vi "test write exist frame.vi"() -> ()   [LabVIEW 2018, in "Data Parser.lvclass"]
uses:
  Data Parser.lvclass
panel:
  out "found":bool
  in  "basic data.move":T1
  in  "frame number":u32
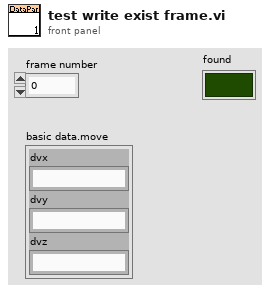
[diagram p1: front panel]
types:
  T1 = cluster{"dvx":string, "dvy":string, "dvz":string}
  T2 = enum16{"open", "replace", "create", "open or create", "replace or create", "replace or create with confirmation"}
  T3 = typedef "Data Parser.lvclass/frame data.ctl" = cluster{"Title":T4, "Basic Data":T5, "Sound":string, "<o> Data":T6, "<bp> Data":T7, "<c> Data":T8, "<w> Data":T9, "<i> Data Array":T10[], "<b> Data Array":T11[]}
  T4 = typedef "Data Parser.lvclass/frame title.ctl" = cluster{"Number":string, "Name":string}
  T5 = typedef "Data Parser.lvclass/frame basic data.ctl" = cluster{"Basic":cluster{"pic":string, "state":string, "wait":string, "next":string}, "Move":cluster{"dvx":string, "dvy":string, "dvz":string}, "Pic Center":cluster{"centerx":string, "centery":string}, "Skill":cluster{"hit_a":string, "hit_d":string, "hit_j":string, "hit_Fa":string, "hit_Ua":string, "hit_Da":string, "hit_Fj":string, "hit_Uj":string, "hit_Dj":string, "hit_ja":string}, "Mp":string}
  T6 = typedef "Data Parser.lvclass/frame o data.ctl" = cluster{"kind":string, "x":string, "y":string, "action":string, "dvx":string, "dvy":string, "dvz":string, "oid":string, "facing":string}
  T7 = typedef "Data Parser.lvclass/frame bp data.ctl" = cluster{"x":string, "y":string}
  T8 = typedef "Data Parser.lvclass/frame c data.ctl" = cluster{"kind":string, "x":string, "y":string, "injury":string, "cover":string, "vaction":string, "aaction":string, "taction":string, "hurtable":string, "decrease":string, "fronthurtact":string, "backhurtact":string, "dircontrol":string, "throwvx":string, "throwvy":string, "throwvz":string, "throwinjury":string}
  T9 = typedef "Data Parser.lvclass/frame w data.ctl" = cluster{"kind":string, "x":string, "y":string, "weaponact":string, "dvx":string, "dvy":string, "dvz":string, "attacking":string, "cover":string}
  T10 = typedef "Data Parser.lvclass/frame i data.ctl" = cluster{"kind":string, "x":string, "y":string, "w":string, "h":string, "dvx":string, "dvy":string, "dvz":string, "fall":string, "arest":string, "vrest":string, "bdefend":string, "injury":string, "zwidth":string, "effect":string, "catchingact":string, "caughtact":string}
  T11 = typedef "Data Parser.lvclass/frame b data.ctl" = cluster{"kind":string, "x":string, "y":string, "w":string, "h":string}
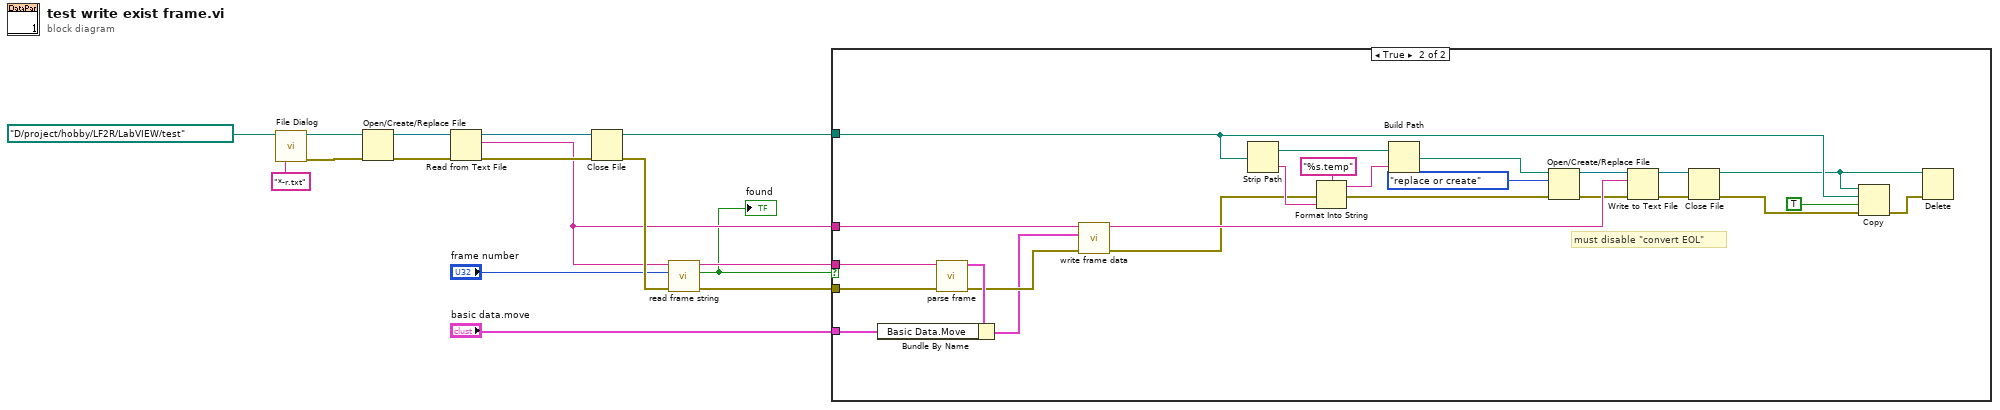
[diagram p0: block diagram]
diagram:
  n1 = call "File Dialog"("start path"=path "D:/project/hobby/LF2R/LabVIEW/test", "pattern (all files)"="*-r.txt") -> ("selected path"=w14:path, "error out"=w13:errorcluster)  [unwired: 10 in, 2 out]
  n2 = Open/Create/Replace File(file path (use dialog)=w14, error in=w13) -> (refnum out=w16:refnum<file>, error out=w15:errorcluster)  [unwired: 4 in, 1 out]
  n3 = Read from Text File(file (use dialog)=w16, error in=w15) -> (refnum out=w7:refnum<file>, text=w3:string, error out=w6:errorcluster)  [unwired: 2 in, 1 out]
  n4 = Close File(refnum=w7, error in=w6) -> (path=w4:path, error out=w5:errorcluster)
  n5 = call "read frame string.vi"("error in"=w5, "frame number"="frame number", "file string"=w3) -> ("error out"=w10:errorcluster, "found"=w1:bool, "<f> string"=w8:string)  [unwired: 5 in, 1 out]
  "found" <- w1
  n6 = case shown="True" w1 {
    tunnel: w10 -> [_ w41]
    tunnel: "basic data.move" -> [_ w39]
    tunnel: w8 -> [_ w38]
    tunnel: w4 -> [_ w37]
    tunnel: w3 -> [_ w36]
    frame False {
    }
    frame True {
      # "must disable \"convert EOL\""
      n7 = call "parse frame.vi"("error in (no error)"=w41, "<f> string"=w38) -> ("error out"=w35:errorcluster, "frame data"=w40:T3)  [unwired: 8 in]
      n8 = Bundle By Name(cluster=w40, "Basic Data.Move"=w39) -> (w17:T3)
      n9 = call "write frame data.vi"("error in"=w35, "frame data"=w17, "file string in"=w36) -> ("error out"=w18:errorcluster, "file string out"=w34:string)  [unwired: 7 in]
      n10 = Strip Path(path=w37) -> (stripped path=w29:path, name=w28:string)
      n11 = Format Into String(format string="%s.temp", error in=w18, w28) -> (resulting string=w26:string, error out=w24:errorcluster)  [unwired: 1 in]
      n12 = Build Path(base path=w29, name or relative path=w26) -> (appended path=w25:path)
      n13 = Open/Create/Replace File(file path (use dialog)=w25, error in=w24, operation (0:open)=T2."replace or create") -> (refnum out=w33:refnum<file>, error out=w32:errorcluster)  [unwired: 3 in, 1 out]
      n14 = Write to Text File(file (use dialog)=w33, text=w34, error in=w32) -> (refnum out=w31:refnum<file>, error out=w30:errorcluster)  [unwired: 1 in, 1 out]
      n15 = Close File(refnum=w31, error in=w30) -> (path=w19:path, error out=w23:errorcluster)
      n16 = Copy(8:w23, 9:TRUE ("overwrite (F)"), 10:w37, 11:w19) -> (0:w21:errorcluster)  [unwired: 1 in, 2 out]
      n17 = Delete(path (use dialog)=w19, error in=w21) -> ()  [unwired: 3 in, 3 out]
    }
  }
